vi "IPI_OptionChangeString.vi"(11 "Options":T3={"Search Direction"=2, "Edge Options"={"Edge Polarity"=1, "Kernel Size"=3, "Width"=1, "Minimum Edge Strength"=21.0, "Interpolation Type"=enum."Bilinear Fixed", "Data Processing Method"=enum."Average"}} {"Search Direction" items=["Left to Right", "Right to Left", "Top to Bottom", "Bottom to Top"]; "Edge Options"."Edge Polarity" items=["All Edges", "Rising Edges", "Falling Edges"]; "Edge Options"."Minimum Edge Strength" format="%.2f"; "Edge Options"."Width" step=2; "Edge Options"."Kernel Size" step=2}) -> (3 "string":string)   [LabVIEW 2015]
uses:
  <vilib>/vision/Measure.llb/Edge Options.ctl
  <vilib>/vision/Measure.llb/Edge Polarity.ctl
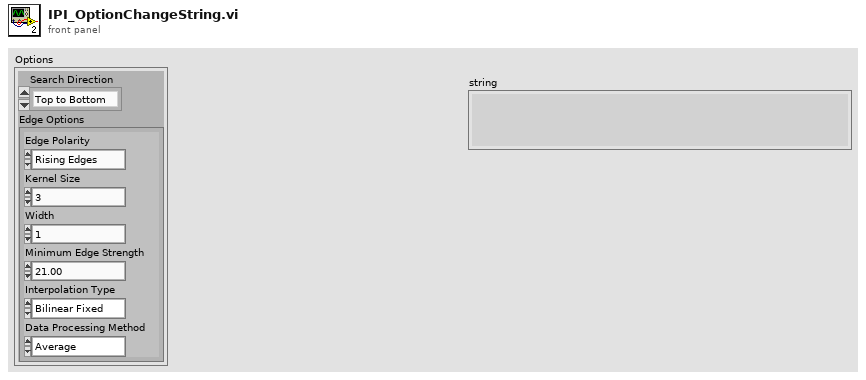
[diagram p1: front panel]
types:
  T1 = typedef "Edge Options.ctl" = cluster{"Edge Polarity":T2, "Kernel Size":u32, "Width":u32, "Minimum Edge Strength":sgl, "Interpolation Type":enum32{"Zero Order", "Bilinear", "Quadratic", "Cubic", "Bilinear Fixed"}, "Data Processing Method":enum32{"Average", "Median"}}
  T2 = typedef "Edge Polarity.ctl" = u32
  T3 = cluster{"Search Direction":u32, "Edge Options":T1}
  T4 = cluster{"Search Direction":u32, "Edge Options":T1, "Show Search Area":bool, "Show Search Lines":bool, "Show Edges Found":bool, "Show Result":bool, "Search Area Color":u32, "Search Lines Color":u32, "Edge Locations Color":u32, "Result Color":u32, "Overlay Group Name":string}
  T5 = enum32{"Zero Order", "Bilinear", "Quadratic", "Cubic", "Bilinear Fixed"}
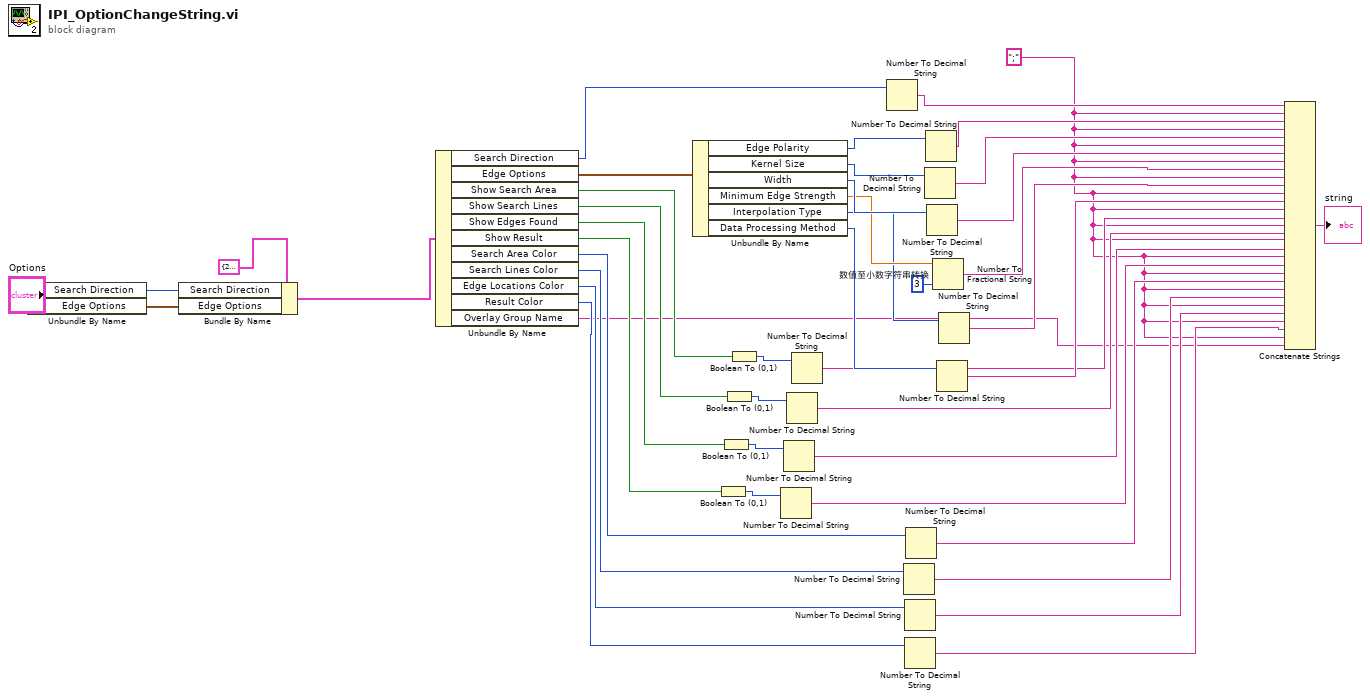
[diagram p0: block diagram]
diagram:
  w8 = ";"
  n1 = Unbundle By Name("Options") -> ("Search Direction"=w3:u32, "Edge Options"=w2:T1)
  n2 = Bundle By Name(cluster=T4 {"Search Direction"=2, "Edge Options"={"Edge Polarity"=1, "Kernel Size"=3, "Width"=1, "Minimum Edge Strength"=21.0, "Interpolation Type"=enum."Bilinear Fixed", "Data Processing Method"=enum."Average"}, "Show Search Area"=TRUE, "Show Search Lines"=FALSE, "Show Edges Found"=FALSE, "Show Result"=TRUE, "Search Area Color"=65280, "Search Lines Color"=255, "Edge Locations Color"=16776960, "Result Color"=16711680, "Overlay Group Name"=""} ("Options (Find Straight Edge 2)"), "Search Direction"=w3, "Edge Options"=w2) -> (w1:T4)
  n3 = Unbundle By Name(w1) -> ("Search Direction"=w43:u32, "Edge Options"=w44:T1, "Show Search Area"=w28:bool, "Show Search Lines"=w25:bool, "Show Edges Found"=w23:bool, "Show Result"=w21:bool, "Search Area Color"=w16:u32, "Search Lines Color"=w15:u32, "Edge Locations Color"=w14:u32, "Result Color"=w13:u32, "Overlay Group Name"=w7:string)
  n4 = Unbundle By Name(w44) -> ("Edge Polarity"=w42:T2, "Kernel Size"=w41:u32, "Width"=w40:u32, "Minimum Edge Strength"=w39:sgl, "Interpolation Type"=w37:T5, "Data Processing Method"=w36:enum32{"Average", "Median"})
  n5 = Boolean To (0,1)(Boolean=w21) -> (0, 1=w22:i16)
  n6 = Boolean To (0,1)(Boolean=w23) -> (0, 1=w24:i16)
  n7 = Boolean To (0,1)(Boolean=w25) -> (0, 1=w26:i16)
  n8 = Boolean To (0,1)(Boolean=w28) -> (0, 1=w27:i16)
  n9 = Number To Decimal String(number=w22) -> (decimal integer string=w17:string)  [unwired: 1 in]
  n10 = Number To Decimal String(number=w24) -> (decimal integer string=w18:string)  [unwired: 1 in]
  n11 = Number To Decimal String(number=w26) -> (decimal integer string=w19:string)  [unwired: 1 in]
  n12 = Number To Decimal String(number=w27) -> (decimal integer string=w20:string)  [unwired: 1 in]
  n13 = Number To Decimal String(number=w43) -> (decimal integer string=w35:string)  [unwired: 1 in]
  n14 = Number To Decimal String(number=w15) -> (decimal integer string=w11:string)  [unwired: 1 in]
  n15 = Number To Decimal String(number=w14) -> (decimal integer string=w10:string)  [unwired: 1 in]
  n16 = Number To Decimal String(number=w13) -> (decimal integer string=w9:string)  [unwired: 1 in]
  n17 = Number To Decimal String(number=w16) -> (decimal integer string=w12:string)  [unwired: 1 in]
  n18 = Number To Decimal String(number=w41) -> (decimal integer string=w33:string)  [unwired: 1 in]
  n19 = Number To Decimal String(number=w42) -> (decimal integer string=w34:string)  [unwired: 1 in]
  n20 = Number To Decimal String(number=w40) -> (decimal integer string=w32:string)  [unwired: 1 in]
  n21 = Number To Fractional String "数值至小数字符串转换"(number=w39, precision (6)=i16 3 ("精度(6)")) -> (F-format string=w31:string)  [unwired: 2 in]
  n22 = Number To Decimal String(number=w36) -> (decimal integer string=w29:string)  [unwired: 1 in]
  n23 = Number To Decimal String(number=w37) -> (decimal integer string=w30:string)  [unwired: 1 in]
  n24 = Concatenate Strings(w35, w8, w34, w8, w33, w8, w32, w8, w31, w8, w30, w8, w29, w8, w20, w8, w19, w8, w18, w8, w17, w8, w12, w8, w11, w8, w10, w8, w9, w8, w7) -> (→"string":string)
